vi "onStop.vi"(8 "error in (no error)":errorcluster, 11 "MAUI":refnum<class "SMO.UI.MAUI.lvclass">) -> (0 "error out":errorcluster, 3 "MAUI out":refnum<class "SMO.UI.MAUI.lvclass">)   [LabVIEW 2020, in "SMO.UI.MAUI.lvclass"]
doc: "JKI State Machine Objects (SMO) 1.3.0.56\nJKI - JKI\nCopyright (c) 2017, JKI"
uses:
  SMO.UI.MAUI.lvclass
  <vilib>/Levylab/SMO.UI.Embedded/SMO.UI.Embedded.lvclass
  C:/Program Files (x86)/National Instruments/LabVIEW 2020/vi.lib/JKI/JKI SMO/SMO/SMO.lvclass
  <vilib>/JKI/JKI SMO/SMO.UI/SMO.UI.lvclass
  <vilib>/JKI/JKI SMO/SMO/SMO.lvclass
panel:
  # "For instructions on how to use the JKI State Machine Objects, examples and video tutorials, visit:\nhttp://jki.net/state-machine-objects/\n\nJKI State Machine Objects™\nhttp://jki.net/state-machine-objects/\nCopyright (C) 2005-2015, JKI <info@jki.net>\nALL RIGHTS RESERVED"
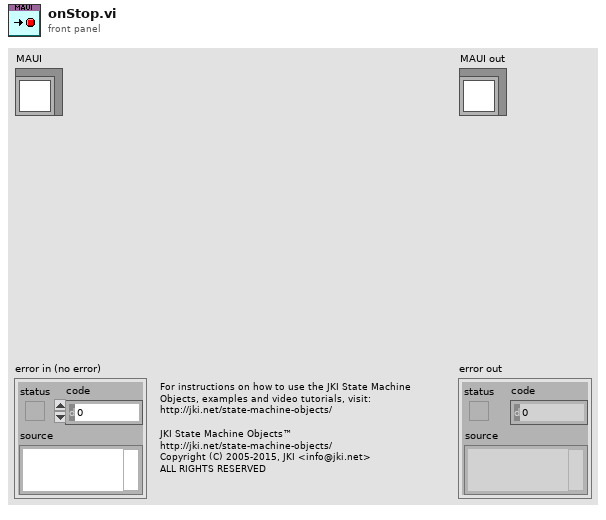
[diagram p1: front panel]
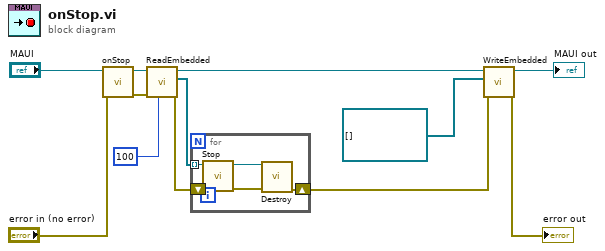
[diagram p0: block diagram]
diagram:
  n1 = call-parent "onStop.vi"("error in (no error)"="error in (no error)", "SMO"="MAUI") -> ("error out"=w2:errorcluster, "SMO out"=w10:refnum<class "SMO.UI.MAUI.lvclass">)  [unwired: 8 in]
  n2 = call "ReadEmbedded.vi"("timeout in ms (-1)"=100, "error in (no error)"=w2, "MAUI in"=w10) -> ("error out"=w8:errorcluster, "Subpanels"=w6:refnum<class "SMO.UI.Embedded.lvclass">[], "MAUI out"=w4:refnum<class "SMO.UI.MAUI.lvclass">)  [unwired: 6 in]
  n3 = for {
    shift-right: [w15] -> w7
    shift-left: w8 -> [w17]
    tunnel: w6 -> [w14] mode=indexing
    n4 = call <vilib>:"Stop.vi"("error in (no error)"=w17, "SMO"=w14) -> ("error out"=w16:errorcluster, "SMO out"=w13:refnum<class "SMO.UI.Embedded.lvclass">)  [unwired: 8 in]
    n5 = call <vilib>:"Destroy.vi"("error in (no error)"=w16, "SMO"=w13) -> ("error out"=w15:errorcluster)  [unwired: 9 in]
  }
  n6 = call "WriteEmbedded.vi"("error in (no error)"=w7, "Subpanels"=refnum<class "SMO.UI.Embedded.lvclass">[] [], "MAUI in"=w4) -> ("error out"=→"error out":errorcluster, "MAUI out"=→"MAUI out":refnum<class "SMO.UI.MAUI.lvclass">)  [unwired: 7 in]
